vi "Write Bottom Right.vi"(8 "error in (no error)":errorcluster, 10 "Bottom Right":cluster{"X":dbl, "Y":dbl}, 11 "Tool Rectangle in":refnum<class "Tool Rectangle.lvclass">) -> (0 "error out":errorcluster, 3 "Tool Rectangle out":refnum<class "Tool Rectangle.lvclass">)   [LabVIEW 2019, in "Tool Rectangle.lvclass"]
uses:
  Tool Rectangle.lvclass
  Tool Rectangle.lvclass/Tool Rectangle.ctl
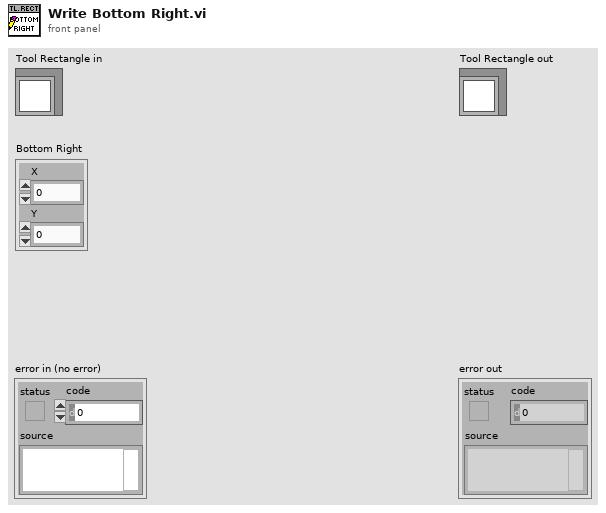
[diagram p1: front panel]
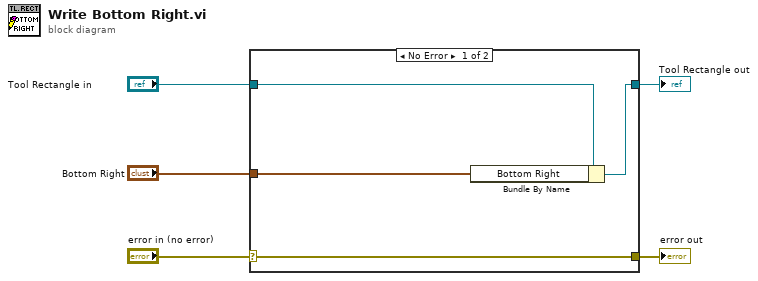
[diagram p0: block diagram]
diagram:
  n1 = case shown="No Error" "error in (no error)" {
    selector: "error in (no error)" -> [w9 w10]
    tunnel: [w9 w10] -> w4
    tunnel: [w7 w11] -> w2
    tunnel: "Tool Rectangle in" -> [w8 w11]
    tunnel: "Bottom Right" -> [w6 _]
    frame No Error {
      n2 = Bundle By Name(cluster=w8, "Bottom Right"=w6) -> (w7:refnum<class "Tool Rectangle.lvclass">)
    }
    frame Error {
    }
  }
  "error out" <- w4
  "Tool Rectangle out" <- w2
